vi "Null Broadcast Events--constant.vi"() -> (3 "NI DAQ Broadcast Events":T1)   [LabVIEW 2020, in "NI DAQ.lvlib"]
doc: "Returns the broadcast events cluster with null references for defining the event types in a Register For Events function.\n_____\nBased on DQMH Project Template 6.1.0.94."
uses:
  NI DAQ.lvlib
  Broadcast Events--cluster.ctl
  Did Init Argument--cluster.ctl
  Status Updated Argument--cluster.ctl
  Error Reported Argument--cluster.ctl
  Stop Argument--cluster.ctl
  Get Module Execution Status Argument--cluster.ctl
  Digital data acquired Argument--cluster.ctl
  Device connected Argument--cluster.ctl
  Connection failed Argument--cluster.ctl
  Analog data acquired Argument--cluster.ctl
  Counter data acquired Argument--cluster.ctl
  Temperature data acquired Argument--cluster.ctl
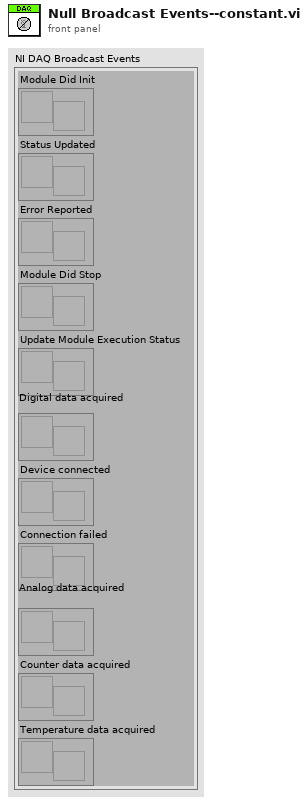
[diagram p1: front panel]
types:
  T1 = typedef "NI DAQ.lvlib/Broadcast Events--cluster.ctl" = cluster{"Module Did Init":refnum<user-event>, "Status Updated":refnum<user-event>, "Error Reported":refnum<user-event>, "Module Did Stop":refnum<user-event>, "Update Module Execution Status":refnum<user-event>, "Digital data acquired":refnum<user-event>, "Device connected":refnum<user-event>, "Connection failed":refnum<user-event>, "Analog data acquired":refnum<user-event>, "Counter data acquired":refnum<user-event>, "Temperature data acquired":refnum<user-event>}
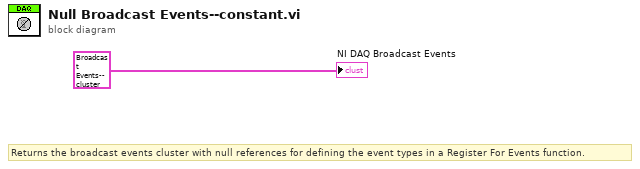
[diagram p0: block diagram]
diagram:
  # "Returns the broadcast events cluster with null references for defining the event types in a Register For Events function."
  "NI DAQ Broadcast Events" <- T1 {"Module Did Init"=refnum, "Status Updated"=refnum, "Error Reported"=refnum, "Module Did Stop"=refnum, "Update Module Execution Status"=refnum, "Digital data acquired"=refnum, "Device connected"=refnum, "Connection failed"=refnum, "Analog data acquired"=refnum, "Counter data acquired"=refnum, "Temperature data acquired"=refnum} ("Broadcast Events")
